vi "my_3rd_vi.vi"() -> ()   [LabVIEW 2019]
panel:
  out "y white":i32[](array[numeric])
  out "x white":i32[](array[numeric])
  out "y yellow":i32[](array[numeric])
  out "x yellow":i32[](array[numeric])
  out "y red":i32[](array[numeric])
  out "x red":i32[](array[numeric])
  out "pos":string
  out "error out":errorcluster
  out "standard error":string
  out "standard output":string
  in  "error in (no error)":errorcluster
  out "Pixmap":u32[](array[numeric])
  out "hauteur":i16
  out "largeur":i16
  out "image":u8[](array[numeric])
  out "image depth":i32
  out "PNG Picture":picture
  in  "Path":path
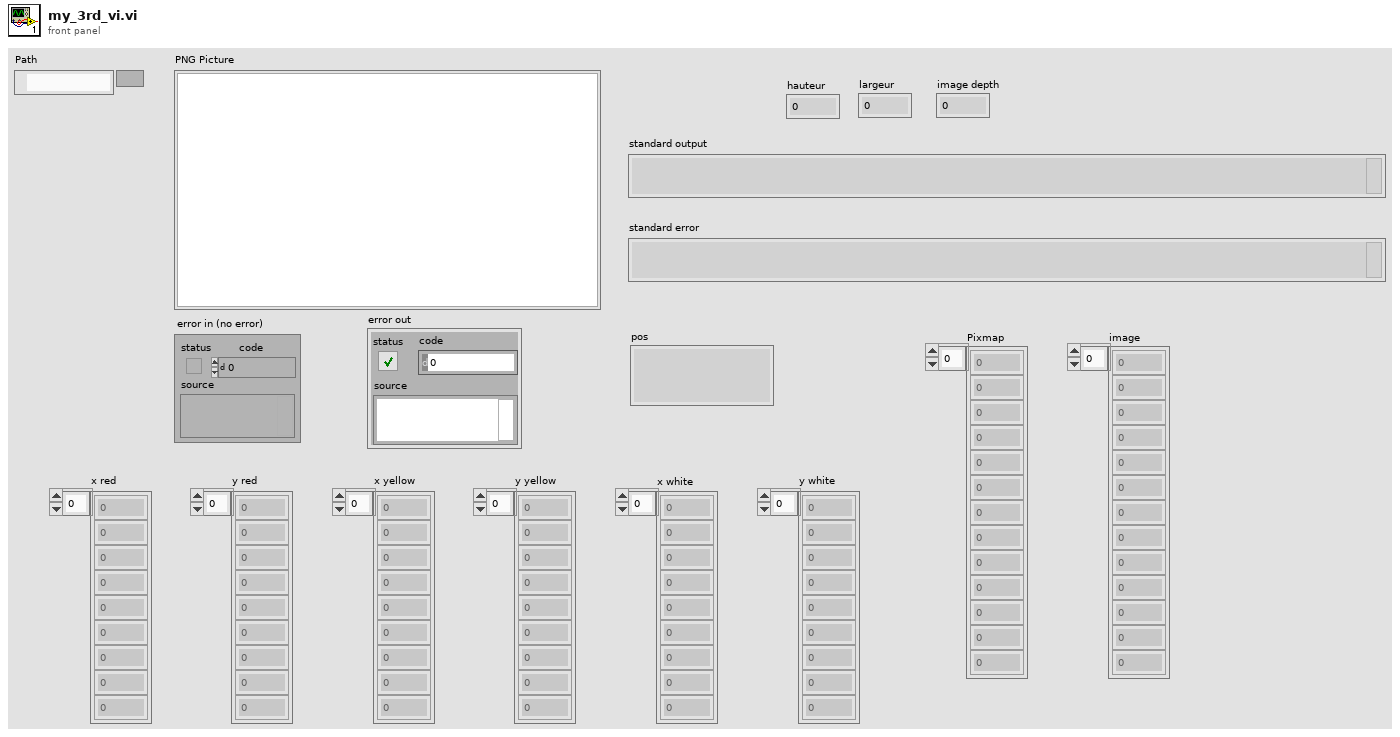
[diagram p1: front panel]
types:
  T1 = cluster{"x red":i32, "y red":i32, "x yellow":i32, "y yellow":i32, "x white":i32, "y white":i32}
  T2 = enum16{"big-endian, network order", "native, host order", "little-endian"}
  T3 = typedef "imagedata.ctl" = cluster{"image type":i32, "image depth":i32, "image":u8[], "mask":u8[], "colors":u32[], "Rectangle":cluster{"left":i16, "top":i16, "right":i16, "bottom":i16}}
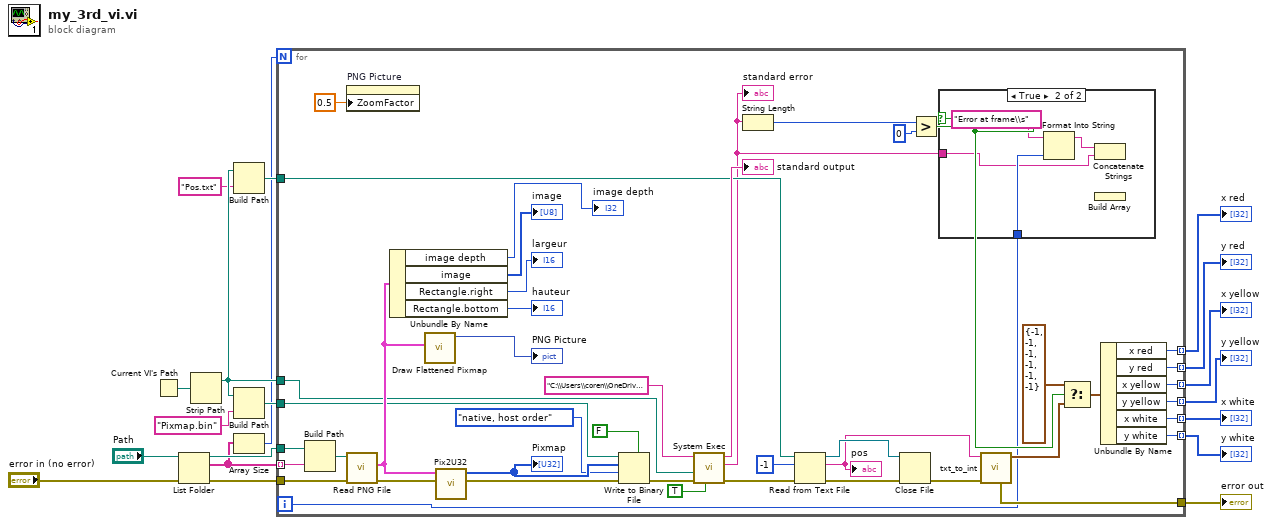
[diagram p0: block diagram]
diagram:
  n1 = Current VI's Path() -> (path=w14:path)
  n2 = List Folder(path="Path", error in="error in (no error)") -> (path out=w17:path, filenames=w8:string[], error out=w15:errorcluster)  [unwired: 2 in, 1 out]
  n3 = Strip Path(path=w14) -> (stripped path=w13:path)  [unwired: 1 out]
  n4 = Build Path(base path=w13, name or relative path="Pos.txt") -> (appended path=w9:path)
  n5 = Build Path(base path=w13, name or relative path="Pixmap.bin") -> (appended path=w11:path)
  n6 = Array Size(array=w8) -> (size(s)=w7:i32)
  n7 = for {
    N: w7 -> [_]
    tunnel: w15 -> [w43]
    tunnel: [w34] -> w19
    tunnel: w17 -> [w42]
    tunnel: w8 -> [w41] mode=indexing
    tunnel: w13 -> [w39]
    tunnel: w11 -> [w38]
    tunnel: w9 -> [w37]
    tunnel: [w33] -> w6 mode=indexing
    tunnel: [w32] -> w5 mode=indexing
    tunnel: [w31] -> w4 mode=indexing
    tunnel: [w30] -> w3 mode=indexing
    tunnel: [w29] -> w2 mode=indexing
    tunnel: [w28] -> w1 mode=indexing
    i -> [w21]
    n8 = Build Path(base path=w42, name or relative path=w41) -> (appended path=w40:path)
    n9 = property on="PNG Picture" class="Pict"("ZoomFactor"=sgl 0.5 ("Zoom Factor")) -> ()  [unwired: 2 in, 2 out]
    n10 = call <vilib>:"Read PNG File.vi"("error in (no error)"=w43, "path to PNG file"=w40) -> ("error out"=w57:errorcluster, "image data"=w52:T3)  [unwired: 7 in, 1 out]
    n11 = Unbundle By Name(w52) -> ("image depth"=→"image depth":i32, "image"=→"image":u8[], "Rectangle.right"=→"largeur":i16, "Rectangle.bottom"=→"hauteur":i16)
    n12 = call <vilib>:"Draw Flattened Pixmap.vi"("image data"=w52) -> ("new picture"=→"PNG Picture":picture)  [unwired: 8 in]
    n13 = call "Pix2U32.vi"("error in (no error)"=w57, "input cluster"=w52) -> ("error out"=w58:errorcluster, "appended array"=w56:u32[])  [unwired: 8 in]
    "Pixmap" <- w56
    n14 = Write to Binary File(file (use dialog)=w38, data=w56, error in=w58, 5:FALSE ("prepend array or string size? (T)"), 9:T2."native, host order" ("byte order (0:big-endian, network order)")) -> (error out=w60:errorcluster)  [unwired: 1 in, 2 out]
    n15 = call <vilib>:"System Exec.vi"("run minimized? (F)"=TRUE, "error in (no error)"=w60, "working directory"=w39, "command line"="C:\\Users\\coren\\OneDrive - epfl.ch\\Documents\\Cours\\prog\\Projet-Billard\\Pix2Pos.exe 98 402 129 748 160 255 0 160 0 160 140 255 140 255 0 175 150 255 150 255 150 255 39 62 91 116 202 255 11") -> ("error out"=w63:errorcluster, "standard error"=w20:string, "standard output"=→"standard output":string)  [unwired: 4 in, 1 out]
    "standard error" <- w20
    n16 = String Length(string=w20) -> (length=w24:i32)
    n17 = Read from Text File(file (use dialog)=w37, count=-1, error in=w63) -> (refnum out=w61:refnum<file>, text=w36:string, error out=w62:errorcluster)  [unwired: 1 in, 1 out]
    "pos" <- w36
    n18 = Close File(refnum=w61, error in=w62) -> (error out=w35:errorcluster)  [unwired: 1 out]
    n19 = Greater?(x=w24, y=0) -> (0:w22:bool)
    n20 = case shown="True" w22 {
      tunnel: w21 -> [_ w67]
      tunnel: w20 -> [_ w65]
      frame False {
      }
      frame True {
        n21 = Format Into String(initial string="Error at frame\\s", w67) -> (resulting string=w66:string)  [unwired: 2 in, 1 out]
        n22 = Concatenate Strings(w66, w65) -> ()  [unwired: 1 out]
        n23 = Build Array() -> (w64:dbl)  [unwired: 1 out]
      }
    }
    n24 = call "txt_to_int.vi"("error in (no error)"=w35, "pos.txt"=w36) -> ("Cluster"=w27:T1, "error out"=w34:errorcluster)  [unwired: 5 in, 3 out]
    n25 = Select(t=T1 {"x red"=-1, "y red"=-1, "x yellow"=-1, "y yellow"=-1, "x white"=-1, "y white"=-1}, s=w22, f=w27) -> (s? t:f=w26:T1)
    n26 = Unbundle By Name(w26) -> ("x red"=w33:i32, "y red"=w32:i32, "x yellow"=w31:i32, "y yellow"=w30:i32, "x white"=w29:i32, "y white"=w28:i32)
  }
  "error out" <- w19
  "x red" <- w6
  "y red" <- w5
  "x yellow" <- w4
  "y yellow" <- w3
  "x white" <- w2
  "y white" <- w1
